vi "PH_Timing.PC Status Interlockswitch.vi"(0 "i ref in":refnum<vi>, 2 "IL Switch Status":T1 items=["no info", "off/false/out", "on/true/in", "Failure", "Alarm", "Status 1", "Status 2", "Status 3"], 3 "no link":bool, 5 "error in":errorcluster) -> (14 "i ref out":refnum<vi>, 19 "error out":errorcluster)   [LabVIEW 2014, in "PH_Timing.lvlib"]
doc: "This VI writes the incoming information to own attributes and sets GUI elements."
uses:
  PH_Timing.lvlib
  PH_StatusHandler/PH_StatusHandler.Status.ctl
  PH_Common/PH_Common.lvlib
  PH_Switch/PH_Switch.lvlib
  PH_StatusHandler/PH_StatusHandler.lvlib
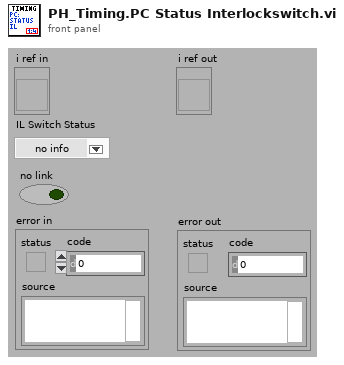
[diagram p1: front panel]
types:
  T1 = typedef "PH_StatusHandler.lvlib/PH_StatusHandler.Status.ctl" = i16
  T2 = typedef "PH_Timing.lvlib/PH_Timing.i attribute.ctl" = cluster{"Sequencer":cluster{"linked?":bool, "Proc State":string, "Ref State":refnum<vi>}, "Gate Generator":cluster{"GD":cluster{"Device Status":T1, "linked?":bool}, "Settings":T3, "GUI Ref":refnum<vi>}, "Interlock Bypass":cluster{"Instancename":string, "Switch linked?":bool, "Device Status":T1, "Ref Status":refnum<vi>}, "Roughtuner":cluster{"Settings":T4, "GUI Ref":refnum<vi>, "GD":cluster{"Device Status":T1, "linked?":bool}}, "0,5Hz Gater":cluster{"Settings":T5, "GUI Ref":refnum<vi>, "GD":cluster{"Device Status":T1, "linked?":bool}}, "Slow Trigger":cluster{"Settings":T6, "GUI Ref":refnum<vi>, "Service ID Delay":i32, "Service ID Ext Trig":i32, "Wanted Settings":T6}, "Timing Mode":cluster{"Mode":T7, "GUI Ref":refnum<vi>, "Service ID T2":i32, "Service ID Mode":i32, "Wanted Mode":T7}, "ns Generator":cluster{"Settings":T8, "ns Generator Settings":refnum<vi>, "GD":cluster{"Device Status":T1, "linked?":bool}}, "Phase FEs":cluster{"Settings":T11, "GUI Ref":refnum<vi>, "Service ID Phase":i32, "Wanted Settings":T11}, "GD GUI Refs":refnum<vi>[], "Heads":T12[], "GUI Ref Delete":refnum<vi>}
  T3 = typedef "PH_Timing.lvlib/PH_Timing.GateGen.ctl" = cluster{"Instance":string, "Channel Gate":i32, "Channel T2":i32, "Width Gate":dbl, "Width T2":dbl, "Delay Gate":dbl, "Delay T2":dbl, "Gate activ":bool, "T2 activ":bool, "System Mode":enum16{"Normal", "Single", "Burst", "Duty Cycle"}}
  T4 = typedef "PH_Timing.lvlib/PH_Timing.Roughtuner.ctl" = cluster{"Instance":string, "Phase PHELIX / UNILAC":cluster{"Channel":u16, "relative to":u16, "Delay [ms]":dbl}, "Pulse Length":cluster{"Channel":u16, "relative to":u16, "Delay [ms]":dbl}, "Trigger":cluster{"externally?":bool, "Rate [Hz]":dbl}}
  T5 = typedef "PH_Timing.lvlib/PH_Timing.0.5HzGater.ctl" = cluster{"Instance":string, "Channel ns FE Delay":i32, "Channel 0.5Hz":i32, "Width ns FE Delay":dbl, "Width 0.5Hz":dbl, "Delay ns FE Delay":dbl, "Delay 0.5Hz":dbl, "ns FE Delay active":bool, "0.5Hz activ":bool, "ns FE Delay inverted":bool, "0.5Hz inverted":bool}
  T6 = typedef "PH_Timing.lvlib/PH_Timing.Slow Trigger Settings.ctl" = cluster{"Delay":dbl, "externally triggered?":bool}
  T7 = typedef "PH_Timing.lvlib/PH_Timing.Timing Mode.ctl" = cluster{"T2":i16, "Modeselector":enum32{"10 Hz", "0.5 Hz", "Shot"}}
  T8 = typedef "PH_Timing.lvlib/PH_Timing.ns Generator.ctl" = cluster{"Instance":string, "Phase fs / ns FE":cluster{"Channel":T9, "Settings":T10}}
  T9 = typedef "Stanford Research DG645 - Driver.lvlib/Channel.ctl" = i32
  T10 = typedef "PH_SRDG645.lvlib/PH_SRDG645.Channel Settings.ctl" = cluster{"Delay [s]":dbl, "relative to":i32}
  T11 = typedef "PH_Timing.lvlib/PH_Timing.Phase FEs.ctl" = cluster{"Phase":dbl}
  T12 = typedef "PH_Timing.lvlib/PH_Timing.PU Data.ctl" = cluster{"linked?":bool, "Data":T13, "GD":cluster{"Device Status":T1, "linked?":bool}, "GUI Ref":refnum<vi>, "PU":T14}
  T13 = typedef "PH_Timing.lvlib/PH_Timing.PU Info.ctl" = cluster{"Act CH?":bool, "GD":string, "CH":i32, "Delay":dbl, "active":bool, "in Use?":bool}
  T14 = typedef "PH_PP_Common.lvlib/PH_PP_Common.PUs.ctl" = enum16{"no Info", "PA-19mm-1", "PA-19mm-2", "PA-45mm-PILC", "PA-45mm-MAIN", "MA-PU-1", "MA-PU-2", "MA-PU-3", "MA-PU-4", "MA-PU-5", "MA-PU-6", "MA-FR", "MA-PILC", "PA-45mm-DP"}
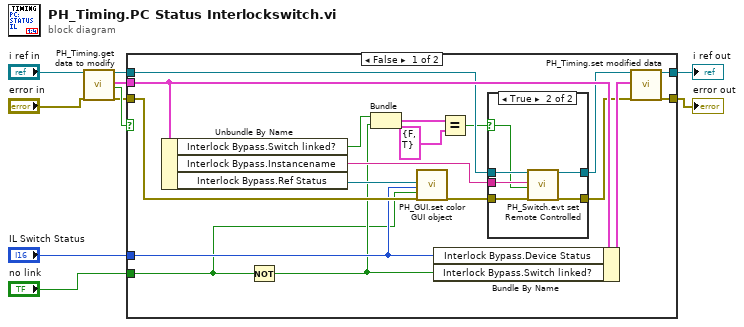
[diagram p0: block diagram]
diagram:
  n1 = call "PH_Timing.get data to modify.vi"("i ref in"="i ref in", "error in (no error)"="error in") -> ("i ref out"=w3:refnum<vi>, "i attribute"=w8:T2, "timed out"=w9:bool, "error out"=w6:errorcluster)  [unwired: 14 in]
  n2 = case shown="False" w9 {
    tunnel: w3 -> [w21 w38]
    tunnel: [w28 w38] -> w4
    tunnel: w6 -> [w24 w37]
    tunnel: [w27 w37] -> w7
    tunnel: w8 -> [w25 _]
    tunnel: "no link" -> [w14 _]
    tunnel: "IL Switch Status" -> [w22 _]
    frame False {
      n3 = Unbundle By Name(w25) -> ("Interlock Bypass.Switch linked?"=w16:bool, "Interlock Bypass.Instancename"=w19:string, "Interlock Bypass.Ref Status"=w23:refnum<vi>)
      n4 = Not(x=w14) -> (.not. x?=w15:bool)
      n5 = Bundle("Switch linked?"=w16, w15) -> (w13:cluster{"Switch linked?":bool, bool})  [unwired: 1 in]
      n6 = call "PH_GUI.set color GUI object.vi"("GUI object Ref"=w23, "State"=w22, "Blinking? (false)"=w14, "error in (no error)"=w24) -> ("error out"=w18:errorcluster)  [unwired: 15 in]
      n7 = Bundle By Name(cluster=w25, "Interlock Bypass.Device Status"=w22, "Interlock Bypass.Switch linked?"=w15) -> (w26:T2)
      n8 = Equal?(x=w13, y=cluster{"linked?":bool, bool} {"linked?"=FALSE, TRUE}) -> (x = y?=w11:bool)
      n9 = case shown="True" w11 {
        selector: w11 -> [_ w31]
        tunnel: w21 -> [w30 w36]
        tunnel: [w30 w35] -> w20
        tunnel: w19 -> [_ w34]
        tunnel: w18 -> [w29 w33]
        tunnel: [w29 w32] -> w17
        frame False {
        }
        frame True {
          n10 = call "PH_Switch.evt set Remote Controlled.vi"("i ref in"=w36, "Instance"=w34, "Remote Controlled"=w31, "error in (no error)"=w33) -> ("i ref out"=w35:refnum<vi>, "error out"=w32:errorcluster)  [unwired: 14 in]
        }
      }
      n11 = call "PH_Timing.set modified data.vi"("i ref in"=w20, "i attribute"=w26, "error in (no error)"=w17) -> ("i ref out"=w28:refnum<vi>, "error out"=w27:errorcluster)  [unwired: 15 in]
    }
    frame True {
    }
  }
  "error out" <- w7
  "i ref out" <- w4
